vi "2. ControlRealTimeACCESS.vi"() -> ()   [LabVIEW 2011]
panel:
  out "Iteration #":i32
  out "mote111":cluster{dbl, dbl}
  out "mote110":cluster{dbl, dbl}
  out "mote109":cluster{dbl, dbl}
  out "mote12":cluster{dbl, dbl}
  out "mote11":cluster{dbl, dbl}
  out "mote8":cluster{dbl, dbl}
  out "mote7":cluster{dbl, dbl}
  out "mote6":cluster{dbl, dbl}
  out "mote5":cluster{dbl, dbl}
  out "mote3":cluster{dbl, dbl}
  out "mote2":cluster{dbl, dbl}
  out "mote4":cluster{dbl, dbl, dbl, dbl}
  out "mote1":cluster{dbl, dbl, dbl, dbl}
  in  "HVAC Testbed":T1(tab)
  out "Motion":bool
  out "CO2":string
  out "Temp":string
  out "Temp":string
  out "CO2":string
  out "Motion":bool
  out "Temp":string
  out "CO2":string
  out "Motion":bool
  out "CO2":string
  out "Temp":string
  out "Motion":bool
  out "Outside temp":dbl(slide) scale=-20.0..40.0
  in  "Heating Valve":u64(slide) scale=0.0..100.0
  in  "Cooling Valve":u64(slide) scale=0.0..100.0
  in  "Fresh Air Valve":u64(slide) scale=0.0..100.0
  out "Temp":string
  out "CO2":string
  out "Motion":bool
  out "CO2":dbl(graph)
  out "Temperature":dbl(graph)
  out "CO2":dbl(graph)
  out "Temperature":dbl(graph)
  in  "Heating Valve":u64(slide) scale=0.0..100.0
  in  "Cooling Valve":u64(slide) scale=0.0..100.0
  in  "Fresh Air Valve":u64(slide) scale=0.0..100.0
  out "Occupancy":dbl
  out "Temp":string
  out "CO2":string
  out "Motion":bool
  out "Light":dbl(slide) scale=0.0..100.0
  in  "12":bool
  in  "11":bool
  in  "4":bool
  in  "111":bool
  in  "110":bool
  in  "109":bool
  in  "8":bool
  in  "7":bool
  in  "5":bool
  in  "4":bool
  in  "3":bool
  in  "1":bool
  in  "6":bool
  in  "2":bool
  out "Humidity":dbl(slide) scale=0.0..100.0
  out "Temperature":dbl(slide) scale=0.0..100.0
  out "CO2 Meter":dbl(knob) scale=0.0..800.0
  out "Selected Mote":string
  out "CO2":dbl(graph)
  out "Temperature":dbl(graph)
  in  "Heating Valve":u64(slide) scale=0.0..100.0
  in  "Cooling Valve":u64(slide) scale=0.0..100.0
  in  "Fresh Air Valve":u64(slide) scale=0.0..100.0
  out "Temp":string
  out "CO2":string
  out "Motion":bool
  in  "HVAC System IP Address":string(combo)="130.237.50.30"
  in  "Password":string
  in  "Username":string
  out "Access to HVAC Msg":errorcluster={"status"=FALSE, "code"=0, "source"="Please Wait ..."}
  # "Actuation"
  # "PLC Data"
  # "Selected Mote Data"
  # "PLC Data"
  # "Actuation"
  # "Actuation"
  # "PLC Data"
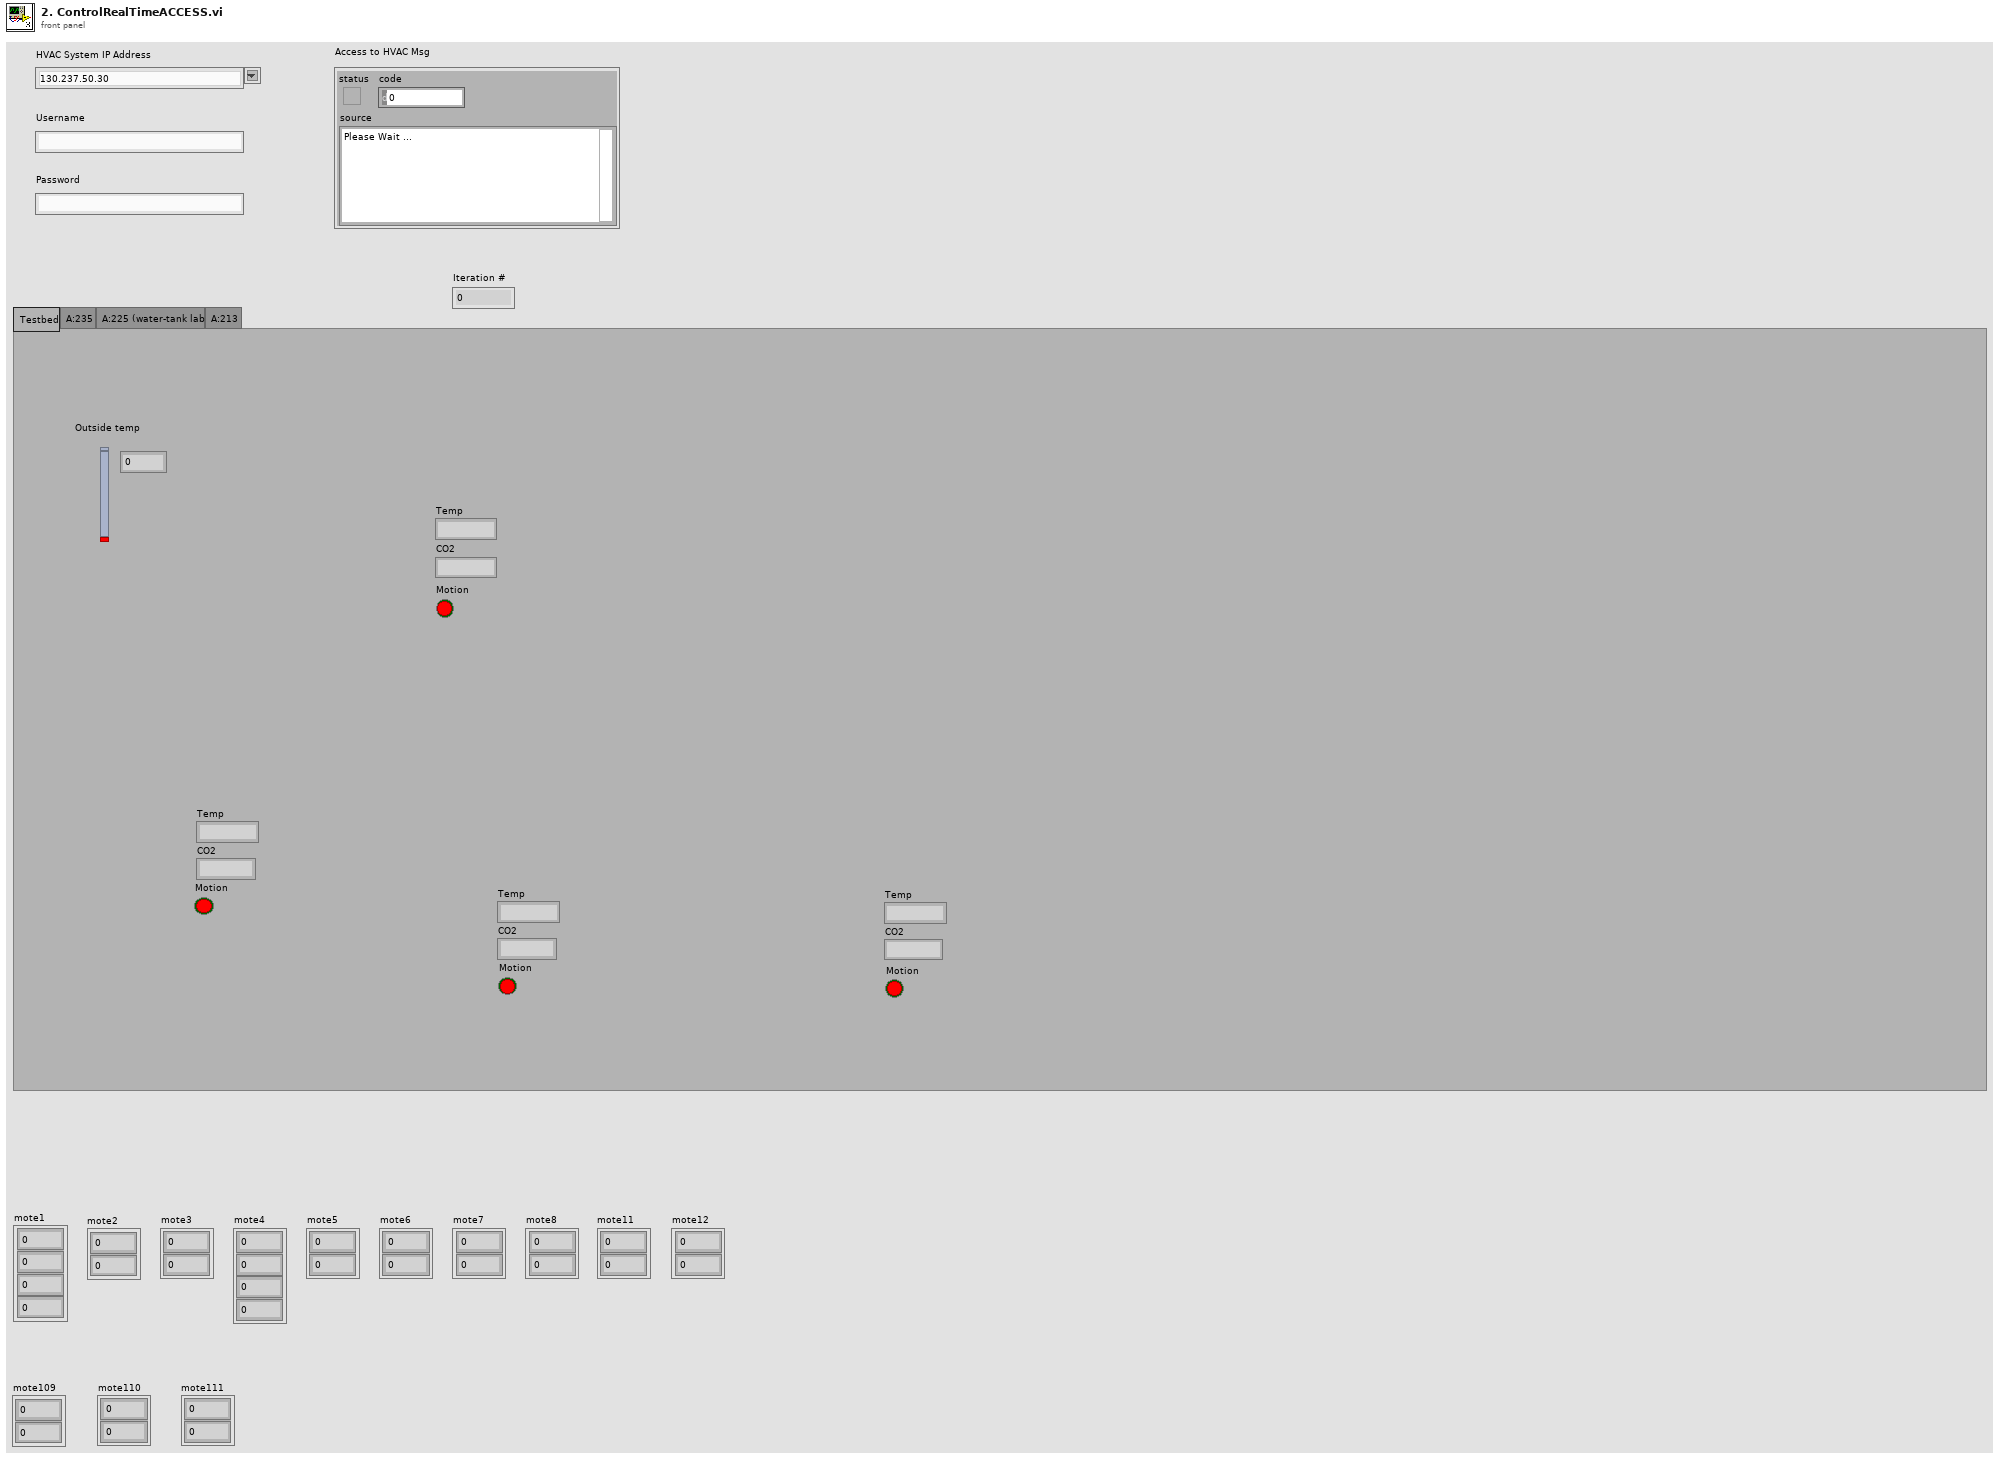
[diagram p1: front panel]
types:
  T1 = enum32{"Testbed", "A:235", "A:225 (water-tank lab)", "A:213"}
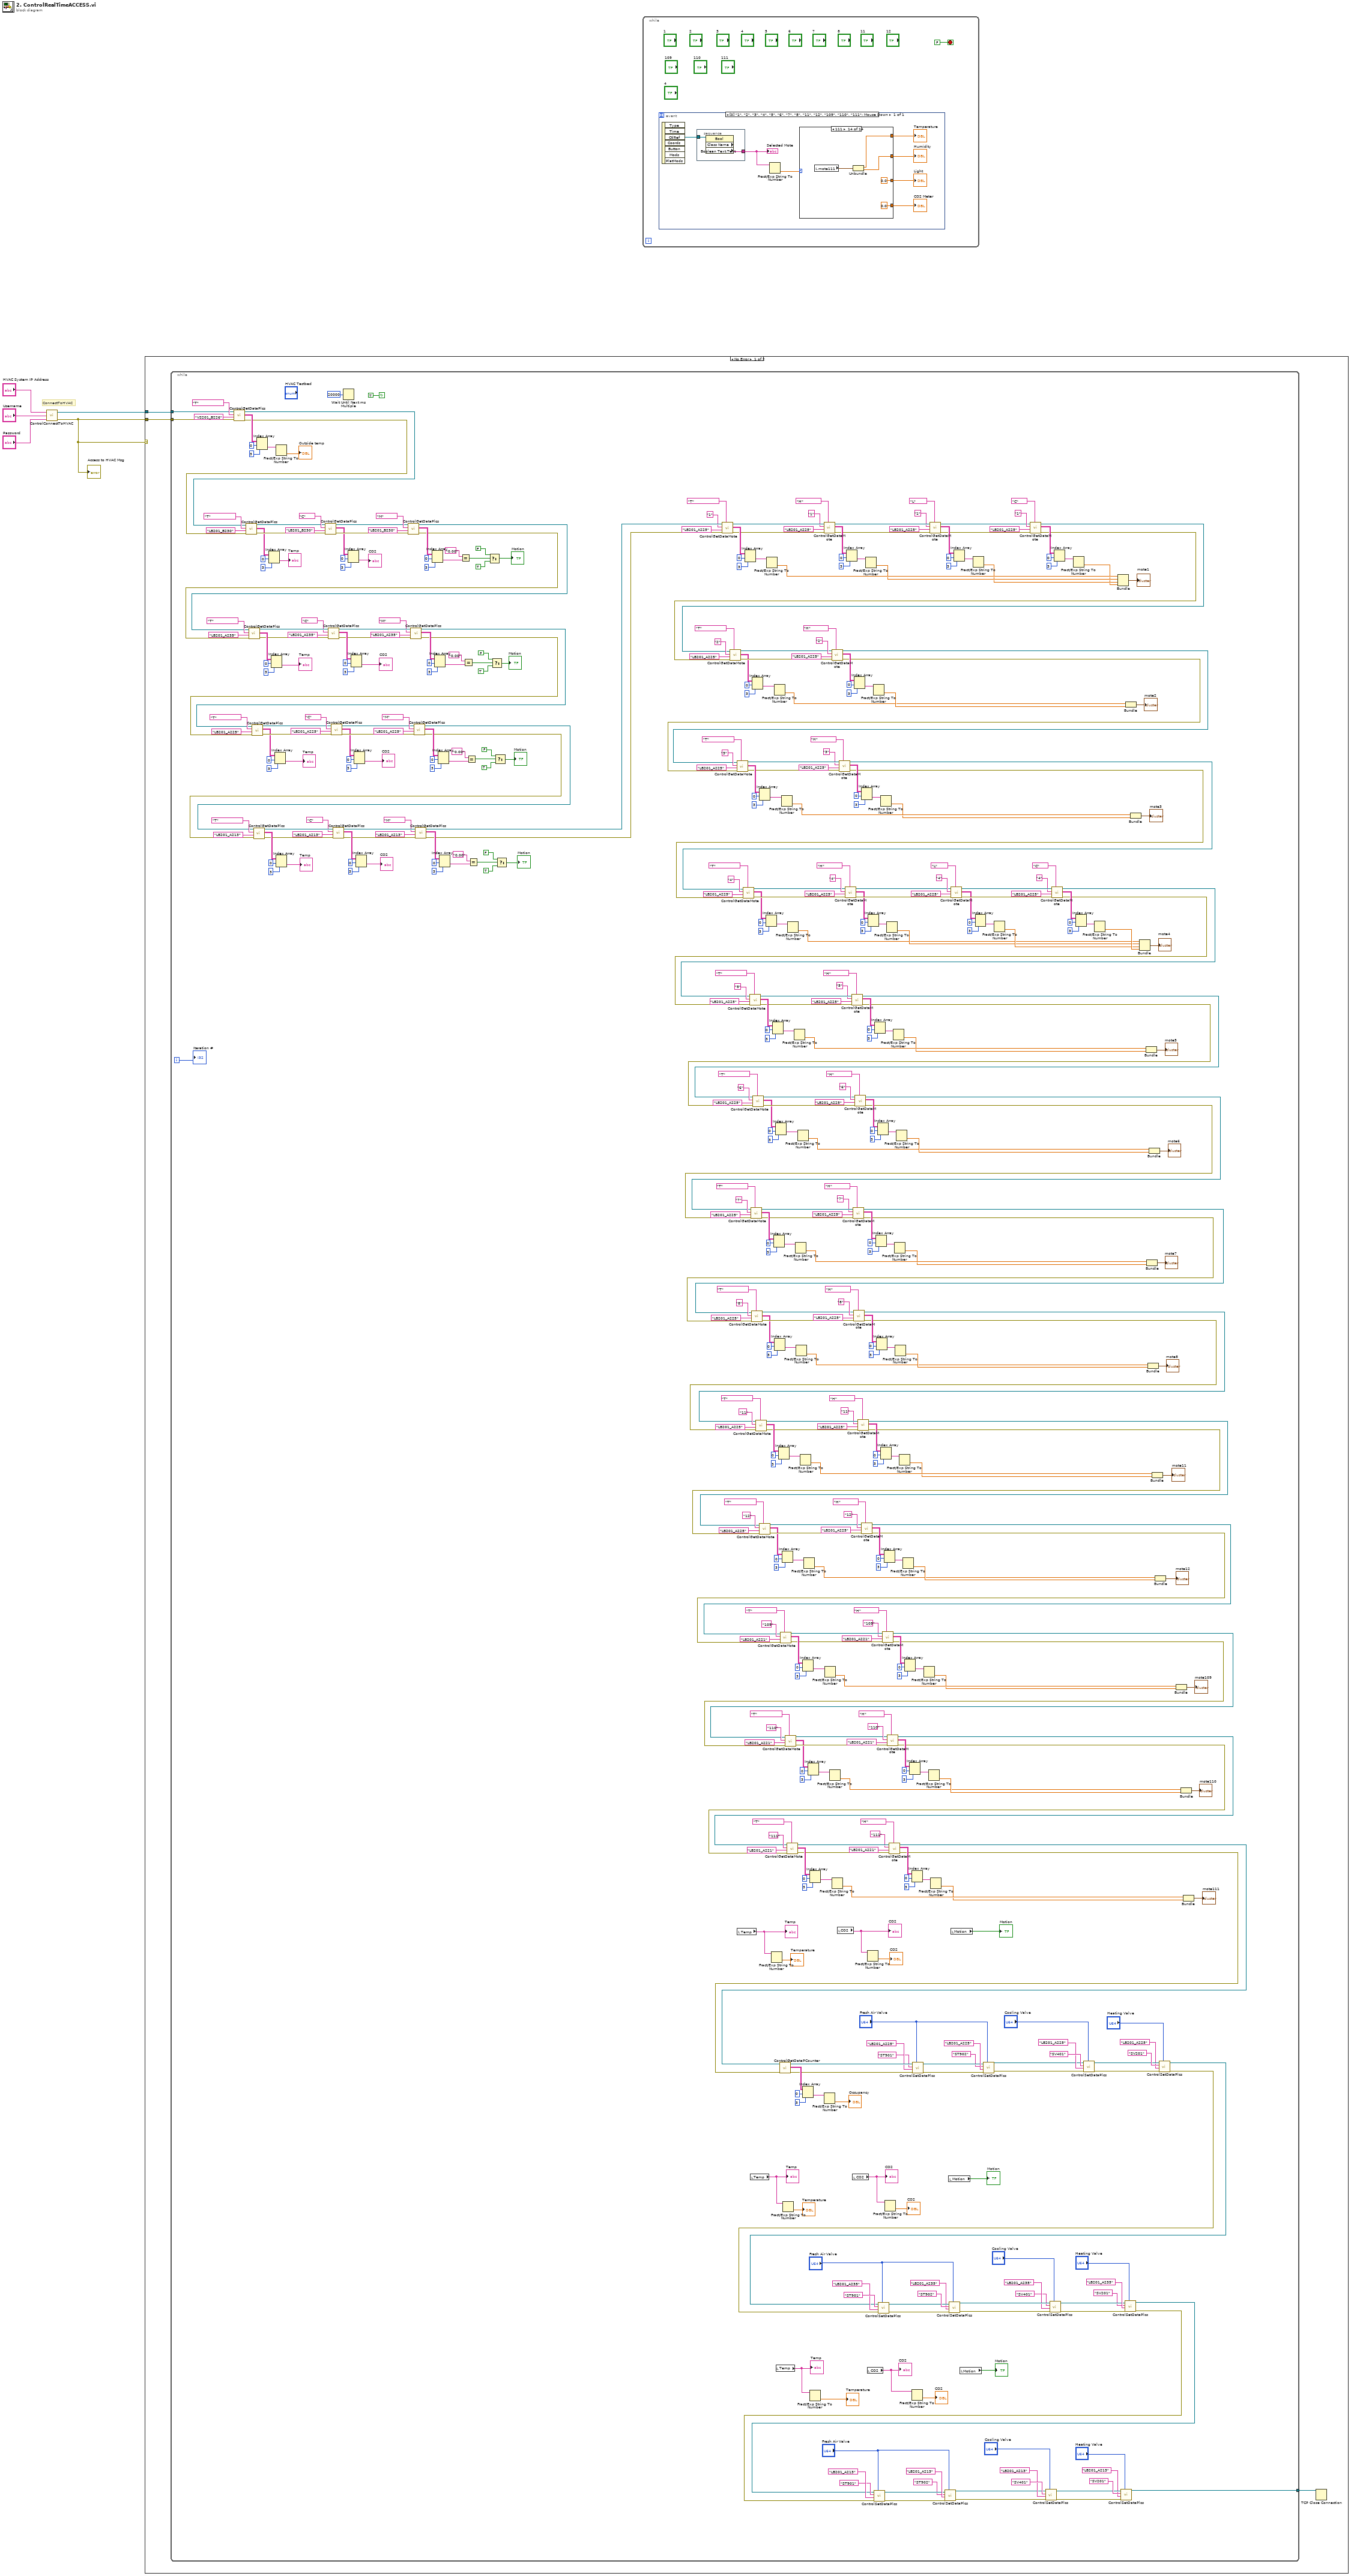
[diagram p0: block diagram]
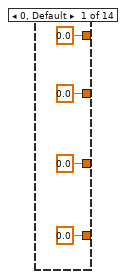
[diagram p2: hidden frame]
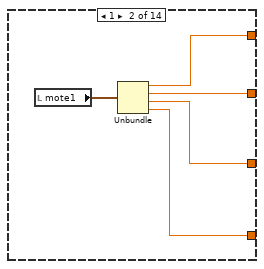
[diagram p3: hidden frame]
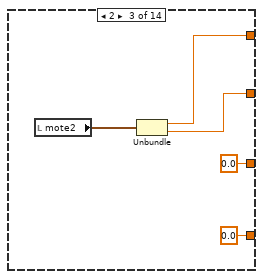
[diagram p4: hidden frame]
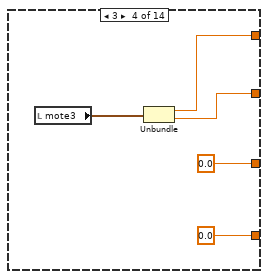
[diagram p5: hidden frame]
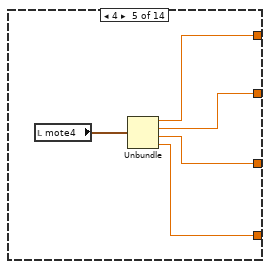
[diagram p6: hidden frame]
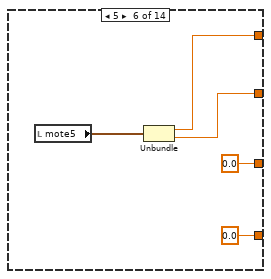
[diagram p7: hidden frame]
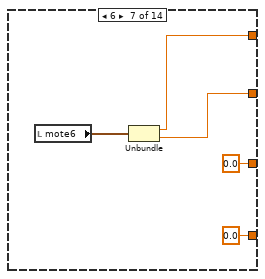
[diagram p8: hidden frame]
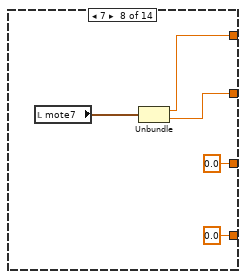
[diagram p9: hidden frame]
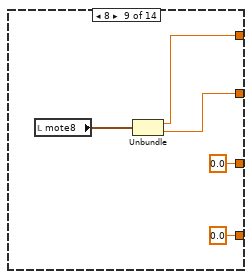
[diagram p10: hidden frame]
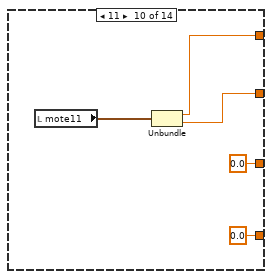
[diagram p11: hidden frame]
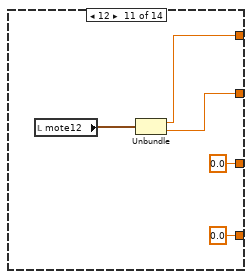
[diagram p12: hidden frame]
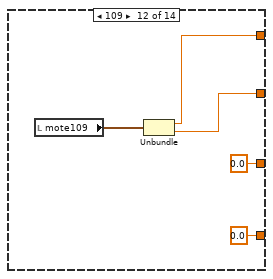
[diagram p13: hidden frame]
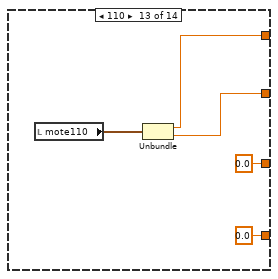
[diagram p14: hidden frame]
diagram:
  # "ConnectToHVAC"
  n1 = call "ControlConnectToHVAC.vi"("Password"="Password", "Username"="Username", "IP Address"="HVAC System IP Address") -> ("error out"=w4:errorcluster, "connection ID out"=w5:refnum<k5>)  [unwired: 1 in]
  "Access to HVAC Msg" <- w4
  n2 = case shown="No Error" w4 {
    tunnel: w5 -> [w7 _]
    tunnel: w4 -> [w8 _]
    frame No Error {
      n3 = while {
        tunnel: w7 -> [w501]
        tunnel: w8 -> [w502]
        tunnel: [w20] -> w6
        i -> [w378]
        stop <- TRUE continue-if-true
        n4 = call "ControlGetDataPlcs.vi"("error in"=w502, "Location"="VS201_B226", "Data Type"="T", "connection ID in"=w501) -> ("error out"=w499:errorcluster, "output array"=w508:string[][], "connection ID out"=w500:refnum<k5>)  [unwired: 4 in]
        n5 = call "ControlGetDataPlcs.vi"("error in"=w499, "Location"="LB201_B230", "Data Type"="T", "connection ID in"=w500) -> ("error out"=w520:errorcluster, "output array"=w515:string[][], "connection ID out"=w521:refnum<k5>)  [unwired: 4 in]
        n6 = Index Array(array=w508, index (row)=0, index (col)=3 ("disabled index (col)")) -> (element=w507:string)
        n7 = Index Array(array=w515, index (row)=0, index (col)=3 ("disabled index (col)")) -> (element=→"Temp":string)
        n8 = Fract/Exp String To Number(string=w507) -> (number=→"Outside temp":dbl)  [unwired: 3 in, 1 out]
        n9 = call "ControlGetDataPlcs.vi"("error in"=w520, "Location"="LB201_B230", "Data Type"="C", "connection ID in"=w521) -> ("error out"=w519:errorcluster, "output array"=w510:string[][], "connection ID out"=w518:refnum<k5>)  [unwired: 4 in]
        n10 = Wait Until Next ms Multiple(millisecond multiple=u32 20000) -> ()  [unwired: 1 out]
        n11 = Index Array(array=w510, index (row)=0, index (col)=3 ("disabled index (col)")) -> (element=→"CO2":string)
        n12 = call "ControlGetDataPlcs.vi"("error in"=w519, "Location"="LB201_B230", "Data Type"="M", "connection ID in"=w518) -> ("error out"=w468:errorcluster, "output array"=w509:string[][], "connection ID out"=w469:refnum<k5>)  [unwired: 4 in]
        n13 = call "ControlGetDataPlcs.vi"("error in"=w468, "Location"="LB201_A235", "Data Type"="T", "connection ID in"=w469) -> ("error out"=w477:errorcluster, "output array"=w482:string[][], "connection ID out"=w476:refnum<k5>)  [unwired: 4 in]
        n14 = Index Array(array=w482, index (row)=0, index (col)=3 ("disabled index (col)")) -> (element=→"Temp":string)
        n15 = call "ControlGetDataPlcs.vi"("error in"=w477, "Location"="LB201_A235", "Data Type"="C", "connection ID in"=w476) -> ("error out"=w478:errorcluster, "output array"=w487:string[][], "connection ID out"=w479:refnum<k5>)  [unwired: 4 in]
        n16 = Index Array(array=w487, index (row)=0, index (col)=3 ("disabled index (col)")) -> (element=→"CO2":string)
        n17 = call "ControlGetDataPlcs.vi"("error in"=w478, "Location"="LB201_A235", "Data Type"="M", "connection ID in"=w479) -> ("error out"=w442:errorcluster, "output array"=w488:string[][], "connection ID out"=w443:refnum<k5>)  [unwired: 4 in]
        n18 = call "ControlGetDataPlcs.vi"("error in"=w442, "Location"="LB201_A225", "Data Type"="T", "connection ID in"=w443) -> ("error out"=w460:errorcluster, "output array"=w455:string[][], "connection ID out"=w461:refnum<k5>)  [unwired: 4 in]
        n19 = Index Array(array=w455, index (row)=0, index (col)=3 ("disabled index (col)")) -> (element=→"Temp":string)
        n20 = call "ControlGetDataPlcs.vi"("error in"=w460, "Location"="LB201_A225", "Data Type"="C", "connection ID in"=w461) -> ("error out"=w459:errorcluster, "output array"=w450:string[][], "connection ID out"=w458:refnum<k5>)  [unwired: 4 in]
        n21 = Index Array(array=w450, index (row)=0, index (col)=3 ("disabled index (col)")) -> (element=→"CO2":string)
        n22 = call "ControlGetDataPlcs.vi"("error in"=w459, "Location"="LB201_A225", "Data Type"="M", "connection ID in"=w458) -> ("error out"=w416:errorcluster, "output array"=w449:string[][], "connection ID out"=w417:refnum<k5>)  [unwired: 4 in]
        n23 = call "ControlGetDataPlcs.vi"("error in"=w416, "Location"="LB201_A213", "Data Type"="T", "connection ID in"=w417) -> ("error out"=w425:errorcluster, "output array"=w430:string[][], "connection ID out"=w424:refnum<k5>)  [unwired: 4 in]
        n24 = Index Array(array=w430, index (row)=0, index (col)=3 ("disabled index (col)")) -> (element=→"Temp":string)
        n25 = call "ControlGetDataPlcs.vi"("error in"=w425, "Location"="LB201_A213", "Data Type"="C", "connection ID in"=w424) -> ("error out"=w426:errorcluster, "output array"=w435:string[][], "connection ID out"=w427:refnum<k5>)  [unwired: 4 in]
        n26 = Index Array(array=w435, index (row)=0, index (col)=3 ("disabled index (col)")) -> (element=→"CO2":string)
        n27 = call "ControlGetDataPlcs.vi"("error in"=w426, "Location"="LB201_A213", "Data Type"="M", "connection ID in"=w427) -> ("error out"=w385:errorcluster, "output array"=w436:string[][], "connection ID out"=w386:refnum<k5>)  [unwired: 4 in]
        n28 = Index Array(array=w509, index (row)=0, index (col)=3 ("disabled index (col)")) -> (element=w497:string)
        n29 = Index Array(array=w488, index (row)=0, index (col)=3 ("disabled index (col)")) -> (element=w490:string)
        n30 = Index Array(array=w449, index (row)=0, index (col)=3 ("disabled index (col)")) -> (element=w447:string)
        n31 = Index Array(array=w436, index (row)=0, index (col)=3 ("disabled index (col)")) -> (element=w438:string)
        n32 = Equal?(x="0,00", y=w497) -> (x = y?=w496:bool)
        n33 = Equal?(x="0,00", y=w490) -> (x = y?=w491:bool)
        n34 = Equal?(x="0,00", y=w447) -> (x = y?=w446:bool)
        n35 = Equal?(x="0,00", y=w438) -> (x = y?=w439:bool)
        n36 = Select(t=FALSE, s=w496, f=TRUE) -> (s? t:f=→"Motion":bool)
        n37 = Select(t=FALSE, s=w491, f=TRUE) -> (s? t:f=→"Motion":bool)
        n38 = Select(t=FALSE, s=w446, f=TRUE) -> (s? t:f=→"Motion":bool)
        n39 = Select(t=FALSE, s=w439, f=TRUE) -> (s? t:f=→"Motion":bool)
        n40 = call "ControlGetDataMote.vi"("Data Type"="T", "error in"=w385, "Location"="LB201_A225", "Node ID"="1", "connection ID in"=w386) -> ("error out"=w391:errorcluster, "output array"=w396:string[][], "connection ID out"=w390:refnum<k5>)  [unwired: 4 in]
        n41 = local read "Temp"() -> (w62:string)
        "Temp" <- w62
        n42 = Index Array(array=w396, index (row)=0, index (col)=3 ("disabled index (col)")) -> (element=w377:string)
        n43 = local read "Temp"() -> (w57:string)
        "Temp" <- w57
        n44 = Fract/Exp String To Number(string=w377) -> (number=w374:dbl)  [unwired: 3 in, 1 out]
        n45 = Fract/Exp String To Number(string=w62) -> (number=→"Temperature":dbl)  [unwired: 3 in, 1 out]
        n46 = local read "Temp"() -> (w38:string)
        "Temp" <- w38
        n47 = Fract/Exp String To Number(string=w57) -> (number=→"Temperature":dbl)  [unwired: 3 in, 1 out]
        n48 = Fract/Exp String To Number(string=w38) -> (number=→"Temperature":dbl)  [unwired: 3 in, 1 out]
        n49 = call "ControlGetDataMote.vi"("Data Type"="H", "error in"=w391, "Location"="LB201_A225", "Node ID"="1", "connection ID in"=w390) -> ("error out"=w392:errorcluster, "output array"=w401:string[][], "connection ID out"=w393:refnum<k5>)  [unwired: 4 in]
        n50 = local read "CO2"() -> (w61:string)
        "CO2" <- w61
        n51 = Index Array(array=w401, index (row)=0, index (col)=3 ("disabled index (col)")) -> (element=w376:string)
        n52 = local read "CO2"() -> (w56:string)
        "CO2" <- w56
        n53 = Fract/Exp String To Number(string=w376) -> (number=w373:dbl)  [unwired: 3 in, 1 out]
        n54 = Fract/Exp String To Number(string=w61) -> (number=→"CO2":dbl)  [unwired: 3 in, 1 out]
        n55 = local read "CO2"() -> (w37:string)
        "CO2" <- w37
        n56 = Fract/Exp String To Number(string=w56) -> (number=→"CO2":dbl)  [unwired: 3 in, 1 out]
        n57 = Fract/Exp String To Number(string=w37) -> (number=→"CO2":dbl)  [unwired: 3 in, 1 out]
        n58 = call "ControlGetDataMote.vi"("Data Type"="L", "error in"=w392, "Location"="LB201_A225", "Node ID"="1", "connection ID in"=w393) -> ("error out"=w361:errorcluster, "output array"=w402:string[][], "connection ID out"=w364:refnum<k5>)  [unwired: 4 in]
        n59 = local read "Motion"() -> (→"Motion":bool)
        n60 = local read "Motion"() -> (→"Motion":bool)
        n61 = Index Array(array=w402, index (row)=0, index (col)=3 ("disabled index (col)")) -> (element=w375:string)
        n62 = local read "Motion"() -> (→"Motion":bool)
        n63 = Fract/Exp String To Number(string=w375) -> (number=w372:dbl)  [unwired: 3 in, 1 out]
        n64 = call "ControlGetDataMote.vi"("Data Type"="C", "error in"=w361, "Location"="LB201_A225", "Node ID"="1", "connection ID in"=w364) -> ("error out"=w284:errorcluster, "output array"=w365:string[][], "connection ID out"=w285:refnum<k5>)  [unwired: 4 in]
        n65 = call "ControlGetDataMote.vi"("Data Type"="T", "error in"=w284, "Location"="LB201_A225", "Node ID"="2", "connection ID in"=w285) -> ("error out"=w349:errorcluster, "output array"=w346:string[][], "connection ID out"=w350:refnum<k5>)  [unwired: 4 in]
        n66 = Index Array(array=w346, index (row)=0, index (col)=3 ("disabled index (col)")) -> (element=w357:string)
        n67 = Fract/Exp String To Number(string=w357) -> (number=w359:dbl)  [unwired: 3 in, 1 out]
        n68 = call "ControlGetDataMote.vi"("Data Type"="H", "error in"=w349, "Location"="LB201_A225", "Node ID"="2", "connection ID in"=w350) -> ("error out"=w280:errorcluster, "output array"=w343:string[][], "connection ID out"=w281:refnum<k5>)  [unwired: 4 in]
        n69 = call "ControlGetDataMote.vi"("Data Type"="T", "error in"=w280, "Location"="LB201_A225", "Node ID"="3", "connection ID in"=w281) -> ("error out"=w336:errorcluster, "output array"=w339:string[][], "connection ID out"=w335:refnum<k5>)  [unwired: 4 in]
        n70 = Index Array(array=w339, index (row)=0, index (col)=3 ("disabled index (col)")) -> (element=w328:string)
        n71 = Fract/Exp String To Number(string=w328) -> (number=w326:dbl)  [unwired: 3 in, 1 out]
        n72 = call "ControlGetDataMote.vi"("Data Type"="H", "error in"=w336, "Location"="LB201_A225", "Node ID"="3", "connection ID in"=w335) -> ("error out"=w282:errorcluster, "output array"=w342:string[][], "connection ID out"=w283:refnum<k5>)  [unwired: 4 in]
        n73 = call "ControlGetDataMote.vi"("Data Type"="T", "error in"=w282, "Location"="LB201_A225", "Node ID"="4", "connection ID in"=w283) -> ("error out"=w297:errorcluster, "output array"=w292:string[][], "connection ID out"=w298:refnum<k5>)  [unwired: 4 in]
        n74 = Index Array(array=w292, index (row)=0, index (col)=3 ("disabled index (col)")) -> (element=w308:string)
        n75 = Fract/Exp String To Number(string=w308) -> (number=w311:dbl)  [unwired: 3 in, 1 out]
        n76 = call "ControlGetDataMote.vi"("Data Type"="H", "error in"=w297, "Location"="LB201_A225", "Node ID"="4", "connection ID in"=w298) -> ("error out"=w296:errorcluster, "output array"=w287:string[][], "connection ID out"=w295:refnum<k5>)  [unwired: 4 in]
        n77 = Index Array(array=w343, index (row)=0, index (col)=3 ("disabled index (col)")) -> (element=w358:string)
        n78 = Index Array(array=w342, index (row)=0, index (col)=3 ("disabled index (col)")) -> (element=w327:string)
        n79 = Index Array(array=w287, index (row)=0, index (col)=3 ("disabled index (col)")) -> (element=w309:string)
        n80 = Fract/Exp String To Number(string=w358) -> (number=w360:dbl)  [unwired: 3 in, 1 out]
        n81 = Fract/Exp String To Number(string=w327) -> (number=w325:dbl)  [unwired: 3 in, 1 out]
        n82 = Fract/Exp String To Number(string=w309) -> (number=w312:dbl)  [unwired: 3 in, 1 out]
        n83 = call "ControlGetDataMote.vi"("Data Type"="L", "error in"=w296, "Location"="LB201_A225", "Node ID"="4", "connection ID in"=w295) -> ("error out"=w324:errorcluster, "output array"=w286:string[][], "connection ID out"=w321:refnum<k5>)  [unwired: 4 in]
        n84 = Index Array(array=w286, index (row)=0, index (col)=3 ("disabled index (col)")) -> (element=w310:string)
        n85 = Fract/Exp String To Number(string=w310) -> (number=w313:dbl)  [unwired: 3 in, 1 out]
        n86 = call "ControlGetDataMote.vi"("Data Type"="C", "error in"=w324, "Location"="LB201_A225", "Node ID"="4", "connection ID in"=w321) -> ("error out"=w168:errorcluster, "output array"=w320:string[][], "connection ID out"=w169:refnum<k5>)  [unwired: 4 in]
        n87 = call "ControlGetDataMote.vi"("Data Type"="T", "error in"=w168, "Location"="LB201_A225", "Node ID"="5", "connection ID in"=w169) -> ("error out"=w271:errorcluster, "output array"=w274:string[][], "connection ID out"=w270:refnum<k5>)  [unwired: 4 in]
        n88 = Index Array(array=w274, index (row)=0, index (col)=3 ("disabled index (col)")) -> (element=w263:string)
        n89 = Fract/Exp String To Number(string=w263) -> (number=w261:dbl)  [unwired: 3 in, 1 out]
        n90 = call "ControlGetDataMote.vi"("Data Type"="H", "error in"=w271, "Location"="LB201_A225", "Node ID"="5", "connection ID in"=w270) -> ("error out"=w164:errorcluster, "output array"=w277:string[][], "connection ID out"=w165:refnum<k5>)  [unwired: 4 in]
        n91 = call "ControlGetDataMote.vi"("Data Type"="T", "error in"=w164, "Location"="LB201_A225", "Node ID"="6", "connection ID in"=w165) -> ("error out"=w248:errorcluster, "output array"=w245:string[][], "connection ID out"=w249:refnum<k5>)  [unwired: 4 in]
        n92 = Index Array(array=w245, index (row)=0, index (col)=3 ("disabled index (col)")) -> (element=w256:string)
        n93 = Fract/Exp String To Number(string=w256) -> (number=w258:dbl)  [unwired: 3 in, 1 out]
        n94 = call "ControlGetDataMote.vi"("Data Type"="H", "error in"=w248, "Location"="LB201_A225", "Node ID"="6", "connection ID in"=w249) -> ("error out"=w161:errorcluster, "output array"=w242:string[][], "connection ID out"=w162:refnum<k5>)  [unwired: 4 in]
        n95 = call "ControlGetDataMote.vi"("Data Type"="T", "error in"=w161, "Location"="LB201_A225", "Node ID"="7", "connection ID in"=w162) -> ("error out"=w235:errorcluster, "output array"=w238:string[][], "connection ID out"=w234:refnum<k5>)  [unwired: 4 in]
        n96 = Index Array(array=w238, index (row)=0, index (col)=3 ("disabled index (col)")) -> (element=w227:string)
        n97 = Fract/Exp String To Number(string=w227) -> (number=w225:dbl)  [unwired: 3 in, 1 out]
        n98 = call "ControlGetDataMote.vi"("Data Type"="H", "error in"=w235, "Location"="LB201_A225", "Node ID"="7", "connection ID in"=w234) -> ("error out"=w158:errorcluster, "output array"=w241:string[][], "connection ID out"=w159:refnum<k5>)  [unwired: 4 in]
        n99 = call "ControlGetDataMote.vi"("Data Type"="T", "error in"=w158, "Location"="LB201_A225", "Node ID"="8", "connection ID in"=w159) -> ("error out"=w212:errorcluster, "output array"=w209:string[][], "connection ID out"=w213:refnum<k5>)  [unwired: 4 in]
        n100 = Index Array(array=w209, index (row)=0, index (col)=3 ("disabled index (col)")) -> (element=w220:string)
        n101 = Fract/Exp String To Number(string=w220) -> (number=w222:dbl)  [unwired: 3 in, 1 out]
        n102 = call "ControlGetDataMote.vi"("Data Type"="H", "error in"=w212, "Location"="LB201_A225", "Node ID"="8", "connection ID in"=w213) -> ("error out"=w118:errorcluster, "output array"=w206:string[][], "connection ID out"=w119:refnum<k5>)  [unwired: 4 in]
        n103 = call "ControlGetDataMote.vi"("Data Type"="T", "error in"=w118, "Location"="LB201_A225", "Node ID"="11", "connection ID in"=w119) -> ("error out"=w199:errorcluster, "output array"=w202:string[][], "connection ID out"=w198:refnum<k5>)  [unwired: 4 in]
        n104 = Index Array(array=w202, index (row)=0, index (col)=3 ("disabled index (col)")) -> (element=w191:string)
        n105 = Fract/Exp String To Number(string=w191) -> (number=w189:dbl)  [unwired: 3 in, 1 out]
        n106 = call "ControlGetDataMote.vi"("Data Type"="H", "error in"=w199, "Location"="LB201_A225", "Node ID"="11", "connection ID in"=w198) -> ("error out"=w116:errorcluster, "output array"=w205:string[][], "connection ID out"=w117:refnum<k5>)  [unwired: 4 in]
        n107 = call "ControlGetDataMote.vi"("Data Type"="T", "error in"=w116, "Location"="LB201_A225", "Node ID"="12", "connection ID in"=w117) -> ("error out"=w176:errorcluster, "output array"=w173:string[][], "connection ID out"=w177:refnum<k5>)  [unwired: 4 in]
        n108 = Index Array(array=w173, index (row)=0, index (col)=3 ("disabled index (col)")) -> (element=w184:string)
        n109 = Fract/Exp String To Number(string=w184) -> (number=w186:dbl)  [unwired: 3 in, 1 out]
        n110 = call "ControlGetDataMote.vi"("Data Type"="H", "error in"=w176, "Location"="LB201_A225", "Node ID"="12", "connection ID in"=w177) -> ("error out"=w93:errorcluster, "output array"=w170:string[][], "connection ID out"=w94:refnum<k5>)  [unwired: 4 in]
        n111 = call "ControlGetDataMote.vi"("Data Type"="T", "error in"=w93, "Location"="LB201_A221", "Node ID"="109", "connection ID in"=w94) -> ("error out"=w151:errorcluster, "output array"=w154:string[][], "connection ID out"=w150:refnum<k5>)  [unwired: 4 in]
        n112 = Index Array(array=w154, index (row)=0, index (col)=3 ("disabled index (col)")) -> (element=w143:string)
        n113 = Fract/Exp String To Number(string=w143) -> (number=w141:dbl)  [unwired: 3 in, 1 out]
        n114 = Index Array(array=w277, index (row)=0, index (col)=3 ("disabled index (col)")) -> (element=w262:string)
        n115 = Index Array(array=w241, index (row)=0, index (col)=3 ("disabled index (col)")) -> (element=w226:string)
        n116 = Index Array(array=w206, index (row)=0, index (col)=3 ("disabled index (col)")) -> (element=w221:string)
        n117 = Index Array(array=w242, index (row)=0, index (col)=3 ("disabled index (col)")) -> (element=w257:string)
        n118 = Index Array(array=w205, index (row)=0, index (col)=3 ("disabled index (col)")) -> (element=w190:string)
        n119 = call "ControlGetDataMote.vi"("Data Type"="H", "error in"=w151, "Location"="LB201_A221", "Node ID"="109", "connection ID in"=w150) -> ("error out"=w91:errorcluster, "output array"=w157:string[][], "connection ID out"=w92:refnum<k5>)  [unwired: 4 in]
        n120 = call "ControlGetDataMote.vi"("Data Type"="T", "error in"=w91, "Location"="LB201_A221", "Node ID"="110", "connection ID in"=w92) -> ("error out"=w128:errorcluster, "output array"=w125:string[][], "connection ID out"=w129:refnum<k5>)  [unwired: 4 in]
        n121 = Index Array(array=w125, index (row)=0, index (col)=3 ("disabled index (col)")) -> (element=w136:string)
        n122 = Fract/Exp String To Number(string=w136) -> (number=w138:dbl)  [unwired: 3 in, 1 out]
        n123 = Index Array(array=w170, index (row)=0, index (col)=3 ("disabled index (col)")) -> (element=w185:string)
        n124 = call "ControlGetDataMote.vi"("Data Type"="H", "error in"=w128, "Location"="LB201_A221", "Node ID"="110", "connection ID in"=w129) -> ("error out"=w89:errorcluster, "output array"=w122:string[][], "connection ID out"=w90:refnum<k5>)  [unwired: 4 in]
        n125 = call "ControlGetDataMote.vi"("Data Type"="T", "error in"=w89, "Location"="LB201_A221", "Node ID"="111", "connection ID in"=w90) -> ("error out"=w109:errorcluster, "output array"=w112:string[][], "connection ID out"=w108:refnum<k5>)  [unwired: 4 in]
        n126 = Index Array(array=w112, index (row)=0, index (col)=3 ("disabled index (col)")) -> (element=w101:string)
        n127 = Fract/Exp String To Number(string=w101) -> (number=w99:dbl)  [unwired: 3 in, 1 out]
        n128 = call "ControlGetDataMote.vi"("Data Type"="H", "error in"=w109, "Location"="LB201_A221", "Node ID"="111", "connection ID in"=w108) -> ("error out"=w83:errorcluster, "output array"=w115:string[][], "connection ID out"=w81:refnum<k5>)  [unwired: 4 in]
        n129 = call "ControlGetDataPCounter.vi"("error in"=w83, "connection ID in"=w81) -> ("error out"=w79:errorcluster, "output array"=w84:string[][], "connection ID out"=w80:refnum<k5>)  [unwired: 7 in]
        n130 = Index Array(array=w84, index (row)=0, index (col)=3 ("disabled index (col)")) -> (element=w87:string)
        n131 = Fract/Exp String To Number(string=w87) -> (number=→"Occupancy":dbl)  [unwired: 3 in, 1 out]
        n132 = Fract/Exp String To Number(string=w262) -> (number=w260:dbl)  [unwired: 3 in, 1 out]
        n133 = Fract/Exp String To Number(string=w226) -> (number=w224:dbl)  [unwired: 3 in, 1 out]
        n134 = Fract/Exp String To Number(string=w221) -> (number=w223:dbl)  [unwired: 3 in, 1 out]
        n135 = Fract/Exp String To Number(string=w257) -> (number=w259:dbl)  [unwired: 3 in, 1 out]
        n136 = Fract/Exp String To Number(string=w190) -> (number=w188:dbl)  [unwired: 3 in, 1 out]
        n137 = Fract/Exp String To Number(string=w185) -> (number=w187:dbl)  [unwired: 3 in, 1 out]
        n138 = Index Array(array=w157, index (row)=0, index (col)=3 ("disabled index (col)")) -> (element=w142:string)
        n139 = Index Array(array=w122, index (row)=0, index (col)=3 ("disabled index (col)")) -> (element=w137:string)
        n140 = Index Array(array=w115, index (row)=0, index (col)=3 ("disabled index (col)")) -> (element=w100:string)
        n141 = call "ControlSetDataPlcs.vi"("data"="Fresh Air Valve", "error in"=w79, "Location"="LB201_A225", "Node ID"="ST901", "connection ID in"=w80) -> ("error out"=w75:errorcluster, "connection ID out"=w76:refnum<k5>)  [unwired: 3 in, 1 out]
        n142 = Fract/Exp String To Number(string=w142) -> (number=w140:dbl)  [unwired: 3 in, 1 out]
        n143 = Fract/Exp String To Number(string=w137) -> (number=w139:dbl)  [unwired: 3 in, 1 out]
        n144 = Fract/Exp String To Number(string=w100) -> (number=w98:dbl)  [unwired: 3 in, 1 out]
        n145 = call "ControlSetDataPlcs.vi"("data"="Fresh Air Valve", "error in"=w75, "Location"="LB201_A225", "Node ID"="ST902", "connection ID in"=w76) -> ("error out"=w65:errorcluster, "connection ID out"=w66:refnum<k5>)  [unwired: 3 in, 1 out]
        n146 = Index Array(array=w365, index (row)=0, index (col)=3 ("disabled index (col)")) -> (element=w371:string)
        n147 = Fract/Exp String To Number(string=w371) -> (number=w363:dbl)  [unwired: 3 in, 1 out]
        n148 = Index Array(array=w320, index (row)=0, index (col)=3 ("disabled index (col)")) -> (element=w314:string)
        n149 = call "ControlSetDataPlcs.vi"("data"="Cooling Valve", "error in"=w65, "Location"="LB201_A225", "Node ID"="SV401", "connection ID in"=w66) -> ("error out"=w70:errorcluster, "connection ID out"=w69:refnum<k5>)  [unwired: 3 in, 1 out]
        n150 = Fract/Exp String To Number(string=w314) -> (number=w322:dbl)  [unwired: 3 in, 1 out]
        n151 = Bundle(w374, w373, w372, w363) -> (→"mote1":cluster{dbl, dbl, dbl, dbl})  [unwired: 1 in]
        n152 = Bundle(w359, w360) -> (→"mote2":cluster{dbl, dbl})  [unwired: 1 in]
        n153 = Bundle(w326, w325) -> (→"mote3":cluster{dbl, dbl})  [unwired: 1 in]
        n154 = Bundle(w311, w312, w313, w322) -> (→"mote4":cluster{dbl, dbl, dbl, dbl})  [unwired: 1 in]
        n155 = Bundle(w261, w260) -> (→"mote5":cluster{dbl, dbl})  [unwired: 1 in]
        n156 = Bundle(w225, w224) -> (→"mote7":cluster{dbl, dbl})  [unwired: 1 in]
        n157 = Bundle(w222, w223) -> (→"mote8":cluster{dbl, dbl})  [unwired: 1 in]
        n158 = Bundle(w258, w259) -> (→"mote6":cluster{dbl, dbl})  [unwired: 1 in]
        n159 = Bundle(w189, w188) -> (→"mote11":cluster{dbl, dbl})  [unwired: 1 in]
        n160 = Bundle(w186, w187) -> (→"mote12":cluster{dbl, dbl})  [unwired: 1 in]
        n161 = call "ControlSetDataPlcs.vi"("data"="Heating Valve", "error in"=w70, "Location"="LB201_A225", "Node ID"="SV201", "connection ID in"=w69) -> ("error out"=w40:errorcluster, "connection ID out"=w41:refnum<k5>)  [unwired: 3 in, 1 out]
        n162 = call "ControlSetDataPlcs.vi"("data"="Fresh Air Valve", "error in"=w40, "Location"="LB201_A235", "Node ID"="ST901", "connection ID in"=w41) -> ("error out"=w45:errorcluster, "connection ID out"=w44:refnum<k5>)  [unwired: 3 in, 1 out]
        n163 = call "ControlSetDataPlcs.vi"("data"="Fresh Air Valve", "error in"=w45, "Location"="LB201_A235", "Node ID"="ST902", "connection ID in"=w44) -> ("error out"=w55:errorcluster, "connection ID out"=w54:refnum<k5>)  [unwired: 3 in, 1 out]
        n164 = call "ControlSetDataPlcs.vi"("data"="Cooling Valve", "error in"=w55, "Location"="LB201_A235", "Node ID"="SV401", "connection ID in"=w54) -> ("error out"=w50:errorcluster, "connection ID out"=w51:refnum<k5>)  [unwired: 3 in, 1 out]
        n165 = call "ControlSetDataPlcs.vi"("data"="Heating Valve", "error in"=w50, "Location"="LB201_A235", "Node ID"="SV201", "connection ID in"=w51) -> ("error out"=w21:errorcluster, "connection ID out"=w22:refnum<k5>)  [unwired: 3 in, 1 out]
        n166 = call "ControlSetDataPlcs.vi"("data"="Fresh Air Valve", "error in"=w21, "Location"="LB201_A213", "Node ID"="ST901", "connection ID in"=w22) -> ("error out"=w33:errorcluster, "connection ID out"=w34:refnum<k5>)  [unwired: 3 in, 1 out]
        n167 = call "ControlSetDataPlcs.vi"("data"="Fresh Air Valve", "error in"=w33, "Location"="LB201_A213", "Node ID"="ST902", "connection ID in"=w34) -> ("error out"=w23:errorcluster, "connection ID out"=w24:refnum<k5>)  [unwired: 3 in, 1 out]
        n168 = call "ControlSetDataPlcs.vi"("data"="Cooling Valve", "error in"=w23, "Location"="LB201_A213", "Node ID"="SV401", "connection ID in"=w24) -> ("error out"=w28:errorcluster, "connection ID out"=w27:refnum<k5>)  [unwired: 3 in, 1 out]
        n169 = call "ControlSetDataPlcs.vi"("data"="Heating Valve", "error in"=w28, "Location"="LB201_A213", "Node ID"="SV201", "connection ID in"=w27) -> ("connection ID out"=w20:refnum<k5>)  [unwired: 3 in, 2 out]
        n170 = Bundle(w141, w140) -> (→"mote109":cluster{dbl, dbl})  [unwired: 1 in]
        n171 = Bundle(w138, w139) -> (→"mote110":cluster{dbl, dbl})  [unwired: 1 in]
        n172 = Bundle(w99, w98) -> (→"mote111":cluster{dbl, dbl})  [unwired: 1 in]
        "Iteration #" <- w378
      }
      n173 = TCP Close Connection(connection ID=w6) -> ()  [unwired: 2 in, 2 out]
    }
    frame Error {
    }
  }
  n174 = while {
    stop <- FALSE stop-if-true
    n175 = event shown="[0] \"1\", \"2\", \"3\", \"4\", \"5\", \"6\", \"7\", \"8\", \"11\", \"12\", \"109\", \"110\", \"111\": Mouse Down" {
      selector: _ -> [_]
      dyn-events: _ -> [_]
      timeout: _ -> [_]
      event "1", "2", "3", "4", "5", "6", "7", "8", "11", "12", "109", "110", "111": Mouse Down {
        n176 = event-data() -> ("CtlRef"=w537:refnum<vi>)  [unwired: 1 in, 6 out]
        n177 = stacked-sequence {
          tunnel: [w608] -> w534
          tunnel: w537 -> [w607]
          frame #0 {
            n178 = property class="Bool" props=["Class Name", "Boolean Text", "Text"](reference=w607) -> ("Boolean Text.Text"=w608:string)  [unwired: 1 in, 3 out]
          }
        }
        "Selected Mote" <- w534
        n179 = Fract/Exp String To Number(string=w534) -> (number=w533:dbl)  [unwired: 3 in, 1 out]
        n180 = case shown="111" w533 {
          tunnel: [0.0 w546 w550 w555 w560 w565 w570 w575 w580 w585 w590 w595 w600 w605] -> w536
          tunnel: [0.0 w545 w549 w554 w559 w564 w569 w574 w579 w584 w589 w594 w599 w604] -> w535
          tunnel: [0.0 w542 0.0 0.0 w557 0.0 0.0 0.0 0.0 0.0 0.0 0.0 0.0 0.0] -> w532
          tunnel: [0.0 w543 0.0 0.0 w558 0.0 0.0 0.0 0.0 0.0 0.0 0.0 0.0 0.0] -> w531
          frame 0, Default {
          }
          frame 1 {
            n181 = local read "mote1"() -> (w544:cluster{dbl, dbl, dbl, dbl})
            n182 = Unbundle(w544) -> (w546:dbl, w545:dbl, w543:dbl, w542:dbl)
          }
          frame 2 {
            n183 = local read "mote2"() -> (w551:cluster{dbl, dbl})
            n184 = Unbundle(w551) -> (w550:dbl, w549:dbl)
          }
          frame 3 {
            n185 = local read "mote3"() -> (w556:cluster{dbl, dbl})
            n186 = Unbundle(w556) -> (w555:dbl, w554:dbl)
          }
          frame 4 {
            n187 = local read "mote4"() -> (w561:cluster{dbl, dbl, dbl, dbl})
            n188 = Unbundle(w561) -> (w560:dbl, w559:dbl, w558:dbl, w557:dbl)
          }
          frame 5 {
            n189 = local read "mote5"() -> (w566:cluster{dbl, dbl})
            n190 = Unbundle(w566) -> (w565:dbl, w564:dbl)
          }
          frame 6 {
            n191 = local read "mote6"() -> (w571:cluster{dbl, dbl})
            n192 = Unbundle(w571) -> (w570:dbl, w569:dbl)
          }
          frame 7 {
            n193 = local read "mote7"() -> (w576:cluster{dbl, dbl})
            n194 = Unbundle(w576) -> (w575:dbl, w574:dbl)
          }
          frame 8 {
            n195 = local read "mote8"() -> (w581:cluster{dbl, dbl})
            n196 = Unbundle(w581) -> (w580:dbl, w579:dbl)
          }
          frame 11 {
            n197 = local read "mote11"() -> (w586:cluster{dbl, dbl})
            n198 = Unbundle(w586) -> (w585:dbl, w584:dbl)
          }
          frame 12 {
            n199 = local read "mote12"() -> (w591:cluster{dbl, dbl})
            n200 = Unbundle(w591) -> (w590:dbl, w589:dbl)
          }
          frame 109 {
            n201 = local read "mote109"() -> (w596:cluster{dbl, dbl})
            n202 = Unbundle(w596) -> (w595:dbl, w594:dbl)
          }
          frame 110 {
            n203 = local read "mote110"() -> (w601:cluster{dbl, dbl})
            n204 = Unbundle(w601) -> (w600:dbl, w599:dbl)
          }
          frame 111 {
            n205 = local read "mote111"() -> (w606:cluster{dbl, dbl})
            n206 = Unbundle(w606) -> (w605:dbl, w604:dbl)
          }
        }
        "Temperature" <- w536
        "Humidity" <- w535
        "CO2 Meter" <- w532
        "Light" <- w531
      }
    }
  }
